vi "CrabWalk_Target.vi"(7 "Speed (m/s)":dbl=0.200707, 8 "error in\n(no error)":errorcluster, 9 "Front Rotate (degree)":dbl, 10 "Distance Y (m)":dbl=0.3, 11 "Distance X (m)":dbl=0.3) -> (0 "error out":errorcluster, 5 "Duration (ms)":dbl)   [LabVIEW 2017]
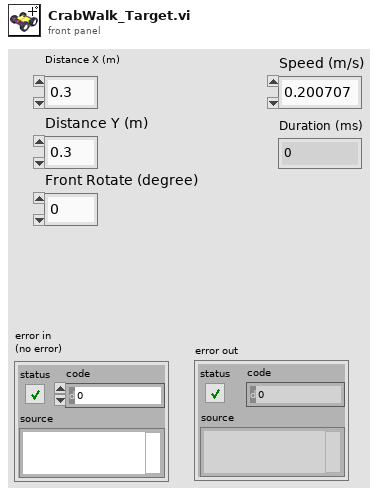
[diagram p1: front panel]
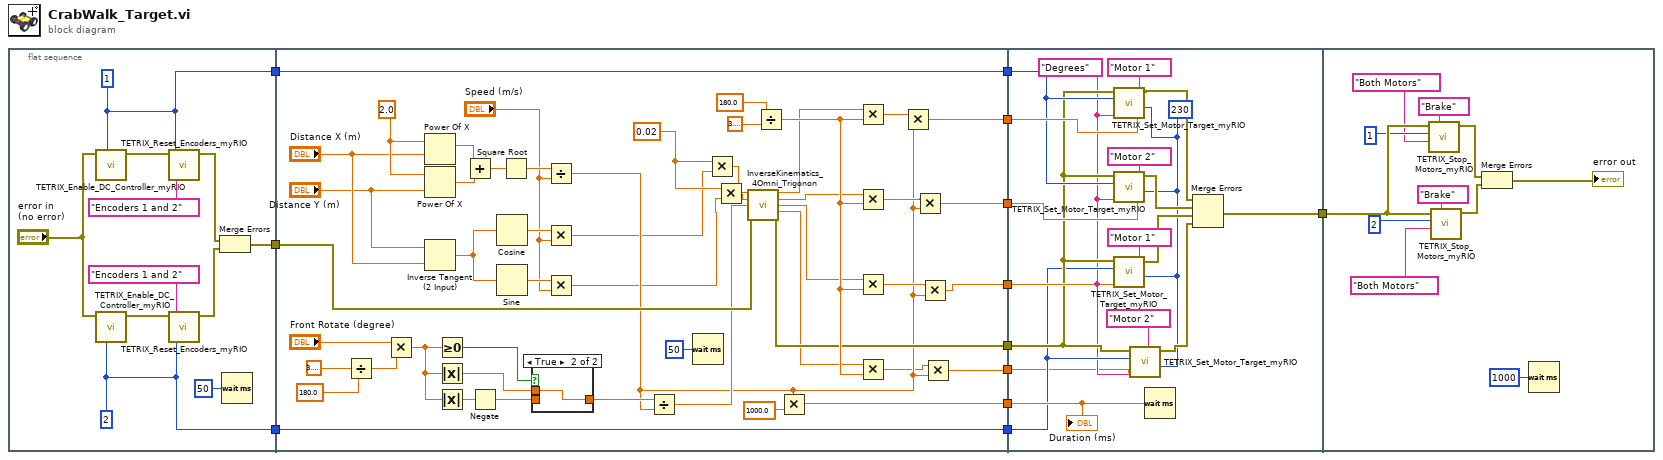
[diagram p0: block diagram]
diagram:
  n1 = flat-sequence {
    tunnel: [w17] -> w12
    tunnel: [w14] -> w11
    tunnel: [w13] -> w10
    tunnel: w12 -> [w45]
    tunnel: w11 -> [w58]
    tunnel: w10 -> [w57]
    tunnel: [w30] -> w9
    tunnel: [w58] -> w8
    tunnel: [w44] -> w7
    tunnel: [w57] -> w6
    tunnel: [w56] -> w5
    tunnel: [w29] -> w4
    tunnel: [w36] -> w3
    tunnel: [w34] -> w2
    tunnel: [w94] -> w1
    tunnel: w9 -> [w77]
    tunnel: w8 -> [w80]
    tunnel: w7 -> [w82]
    tunnel: w6 -> [w88]
    tunnel: w5 -> [w93]
    tunnel: w4 -> [w83]
    tunnel: w3 -> [w91]
    tunnel: w2 -> [w86]
    tunnel: w1 -> [w103]
    frame #0 {
      w13 = u8 1 ("Controller ID#  (I2C Address)")
      w14 = u8 2 ("Controller ID#  (I2C Address)")
      n2 = call <vilib>:"TETRIX_Enable_DC_Controller_myRIO.vi"("Controller ID#  (I2C Address)"=w13, "Error/Flow In"="error in\n(no error)") -> ("Error/Flow Out"=w22:errorcluster)  [unwired: 5 in]
      n3 = call <vilib>:"TETRIX_Enable_DC_Controller_myRIO.vi"("Controller ID#  (I2C Address)"=w14, "Error/Flow In"="error in\n(no error)") -> ("Error/Flow Out"=w23:errorcluster)  [unwired: 5 in]
      n4 = call <vilib>:"TETRIX_Reset_Encoders_myRIO.vi"("Select Encoder"="Encoders 1 and 2", "Controller ID#  (I2C Address)"=w13, "Error/Flow In"=w22) -> ("Error/Flow Out"=w19:errorcluster)  [unwired: 4 in]
      n5 = call <vilib>:"TETRIX_Reset_Encoders_myRIO.vi"("Select Encoder"="Encoders 1 and 2", "Controller ID#  (I2C Address)"=w14, "Error/Flow In"=w23) -> ("Error/Flow Out"=w18:errorcluster)  [unwired: 4 in]
      n6 = Merge Errors(w19, w18) -> (w17:errorcluster)
      n7 = Wait (ms)(milliseconds to wait=u32 50) -> ()  [unwired: 1 out]
    }
    frame #1 {
      w25 = 0.02 ("x")
      w72 = 2.0 ("y")
      n8 = Divide(x=3.141592653589793, y=180.0) -> (x/y=w64:dbl)
      n9 = Multiply(x="Front Rotate (degree)", y=w64) -> (x*y=w47:dbl)
      n10 = Power Of X(1:"Distance X (m)", 2:w72) -> (0:w71:dbl)
      n11 = Power Of X(1:"Distance Y (m)", 2:w72) -> (0:w70:dbl)
      n12 = Inverse Tangent (2 Input)(1:"Distance X (m)", 2:"Distance Y (m)") -> (0:w51:dbl)
      n13 = Greater Or Equal To 0?(x=w47) -> (x >= 0?=w46:bool)
      n14 = Absolute Value(x=w47) -> (abs(x)=w60:dbl)
      n15 = Absolute Value(x=w47) -> (abs(x)=w62:dbl)
      n16 = Add(x=w71, y=w70) -> (x+y=w73:dbl)
      n17 = Negate(x=w62) -> (-x=w61:dbl)
      n18 = Cosine(x=w51) -> (cos(x)=w68:dbl)
      n19 = Sine(x=w51) -> (sin(x)=w67:dbl)
      n20 = Square Root(x=w73) -> (sqrt(x)=w69:dbl)
      n21 = case shown="True" w46 {
        tunnel: w60 -> [_ w75]
        tunnel: w61 -> [w74 _]
        tunnel: [w74 w75] -> w59
        frame False {
        }
        frame True {
        }
      }
      n22 = Divide(x=w69, y="Speed (m/s)") -> (x/y=w32:dbl)
      n23 = Multiply(x=w68, y="Speed (m/s)") -> (x*y=w24:dbl)
      n24 = Multiply(x=w67, y="Speed (m/s)") -> (x*y=w27:dbl)
      n25 = Divide(x=w59, y=w32) -> (x/y=w39:dbl)
      n26 = Wait (ms)(milliseconds to wait=u32 50) -> ()  [unwired: 1 out]
      n27 = Multiply(x=w25, y=w24) -> (x*y=w28:dbl)
      n28 = Multiply(x=w25, y=w27) -> (x*y=w26:dbl)
      n29 = call "InverseKinematics_4Omni_Trigonon.vi"("VX"=w28, "VY"=w26, "Omega"=w39, "error in (no error)"=w45) -> ("W1-FL"=w40:dbl, "W2-BL"=w41:dbl, "W3-FR"=w42:dbl, "W4-BR"=w43:dbl, "error out"=w44:errorcluster)  [unwired: 7 in]
      n30 = Divide(x=180.0, y=3.141592653589793) -> (x/y=w52:dbl)
      n31 = Multiply(x=w32, y=1000.0) -> (x*y=w56:dbl)
      n32 = Multiply(x=w40, y=w52) -> (x*y=w37:dbl)
      n33 = Multiply(x=w41, y=w52) -> (x*y=w35:dbl)
      n34 = Multiply(x=w42, y=w52) -> (x*y=w33:dbl)
      n35 = Multiply(x=w43, y=w52) -> (x*y=w31:dbl)
      n36 = Multiply(x=w37, y=w32) -> (x*y=w36:dbl)
      n37 = Multiply(x=w35, y=w32) -> (x*y=w34:dbl)
      n38 = Multiply(x=w33, y=w32) -> (x*y=w29:dbl)
      n39 = Multiply(x=w31, y=w32) -> (x*y=w30:dbl)
    }
    frame #2 {
      w76 = i16 230 ("Constant Speed (Degrees per Second)")
      w78 = "Degrees" ("Encoder Units")
      n40 = call <vilib>:"TETRIX_Set_Motor_Target_myRIO.vi"("Motor Encoder Target"=w91, "Constant Speed (Degrees per Second)"=w76, "Encoder Units"=w78, "Select Channel"="Motor 1", "Controller ID#  (I2C Address)"=w88, "Error/Flow In"=w82) -> ("Error/Flow Out"=w90:errorcluster)  [unwired: 1 in]
      n41 = call <vilib>:"TETRIX_Set_Motor_Target_myRIO.vi"("Motor Encoder Target"=w86, "Constant Speed (Degrees per Second)"=w76, "Encoder Units"=w78, "Select Channel"="Motor 2", "Controller ID#  (I2C Address)"=w88, "Error/Flow In"=w82) -> ("Error/Flow Out"=w89:errorcluster)  [unwired: 1 in]
      n42 = call <vilib>:"TETRIX_Set_Motor_Target_myRIO.vi"("Motor Encoder Target"=w83, "Constant Speed (Degrees per Second)"=w76, "Encoder Units"=w78, "Select Channel"="Motor 1", "Controller ID#  (I2C Address)"=w80, "Error/Flow In"=w82) -> ("Error/Flow Out"=w85:errorcluster)  [unwired: 1 in]
      n43 = call <vilib>:"TETRIX_Set_Motor_Target_myRIO.vi"("Motor Encoder Target"=w77, "Constant Speed (Degrees per Second)"=w76, "Encoder Units"=w78, "Select Channel"="Motor 2", "Controller ID#  (I2C Address)"=w80, "Error/Flow In"=w82) -> ("Error/Flow Out"=w81:errorcluster)  [unwired: 1 in]
      n44 = Wait (ms)(milliseconds to wait=w93) -> ()  [unwired: 1 out]
      n45 = Merge Errors(w90, w89, w85, w81) -> (w94:errorcluster)
      "Duration (ms)" <- w93
    }
    frame #3 {
      n46 = call <vilib>:"TETRIX_Stop_Motors_myRIO.vi"("Stop Mode"="Brake", "Select Channel"="Both Motors", "Controller ID#  (I2C Address)"=u8 1, "Error/Flow In"=w103) -> ("Error/Flow Out"=w105:errorcluster)  [unwired: 3 in]
      n47 = call <vilib>:"TETRIX_Stop_Motors_myRIO.vi"("Stop Mode"="Brake", "Select Channel"="Both Motors", "Controller ID#  (I2C Address)"=u8 2, "Error/Flow In"=w103) -> ("Error/Flow Out"=w104:errorcluster)  [unwired: 3 in]
      n48 = Merge Errors(w105, w104) -> (→"error out":errorcluster)
      n49 = Wait (ms)(milliseconds to wait=u32 1000) -> ()  [unwired: 1 out]
    }
  }
